vi "Configure Raw Frames RTM.vi"(8 "error in (no error)":errorcluster, 11 "Node Ptr":u64 format="%.0x") -> (0 "error out":errorcluster)   [LabVIEW 2020, in "AIM ARINC 664 System Explorer.lvlib" / "Implementation.lvlib"]
uses:
  Implementation.lvlib
  Frame Configuration/FrameEditor.lvlib
  Scripting/AIM ARINC 664 Scripting.lvlib
  <vilib>/Utility/SystemLogging/NI_SystemLogging.lvlib
  <vilib>/NI VeriStand/Custom Device Tools/Custom Device Utility Library/Custom Device Utility Library.lvlib
  <vilib>/NI VeriStand/Custom Device API/Custom Device API.lvlib
panel:
  in  "Tag":string
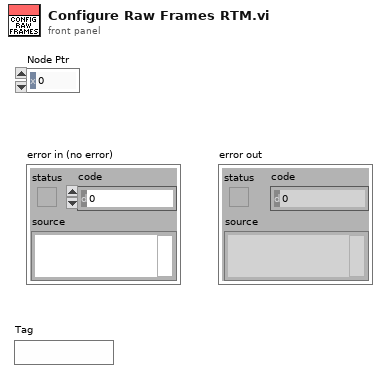
[diagram p1: front panel]
types:
  T1 = typedef "frame_record_type.ctl" = cluster{"HeaderInfo":T2, "Data":u8[]}
  T2 = typedef "AIM664LV.lvlib/queue_header_generic.ctl" = cluster{"InterFrameGap":u32, "PacketGroupWaitTime":u32, "PayloadBufferMode":u8, "PayloadGenerationMode":u8, "PreambleCount":u8, "Skew":u32, "NetSelect":u8, "FrameStartMode":u8, "PhysErrorInjection":u32, "SequenceNumberInit":u16, "SequenceNumberOffset":u16}
  T3 = typedef "Custom Device API.lvlib/Custom Device Item Ref.ctl" = u64
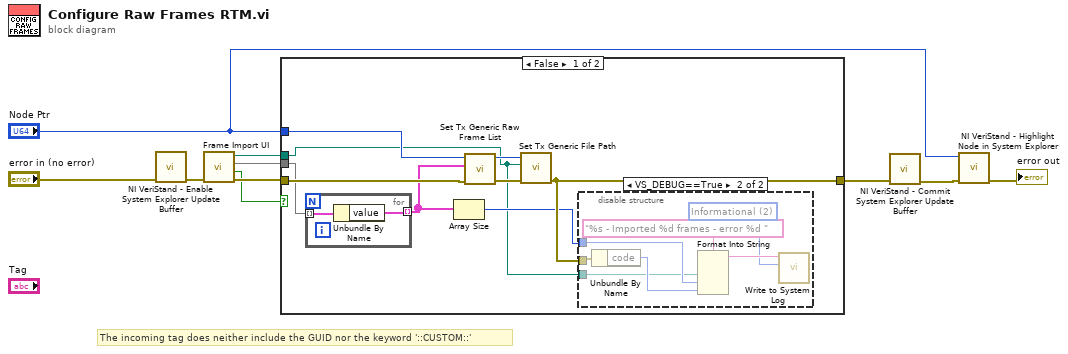
[diagram p0: block diagram]
diagram:
  # "The incoming tag does neither include the GUID nor the keyword '::CUSTOM::'"
  n1 = call <vilib>:"NI VeriStand - Enable System Explorer Update Buffer.vi"("error in (no error)"="error in (no error)") -> ("error out"=w2:errorcluster)  [unwired: 10 in]
  n2 = call "Frame Import UI.vi"("error in"=w2) -> ("error out"=w10:errorcluster, "Cancelled"=w9:bool, "frame map out"=w8:map{string, T1}, "Currently Loaded file"=w7:path)  [unwired: 7 in]
  n3 = case shown="False" w9 {
    tunnel: w10 -> [w16 w29]
    tunnel: [w13 w29] -> w5
    tunnel: "Node Ptr" -> [w18 _]
    tunnel: w8 -> [w15 _]
    tunnel: w7 -> [w11 _]
    frame False {
      n4 = for {
        tunnel: w15 -> [w28] mode=indexing
        tunnel: [w27] -> w14 mode=indexing
        n5 = Unbundle By Name(w28) -> ("value"=w27:T1)
      }
      n6 = Array Size(array=w14) -> (size(s)=w12:i32)
      n7 = call "Set Tx Generic Raw Frame List.vi"("error in"=w16, "Raw Frame List"=w14, "generic tx section in"=w18) -> ("error out"=w19:errorcluster, "generic tx section out"=w17:T3)  [unwired: 7 in]
      n8 = call "Set Tx Generic File Path.vi"("error in"=w19, "Frame Array File Path"=w11, "generic tx section in"=w17) -> ("error out"=w13:errorcluster)  [unwired: 7 in, 1 out]
      n9 = disable-structure shown="VS_DEBUG==True" {
        disable-tunnel: w13 -> [_ w23]
        disable-tunnel: w12 -> [_ w21]
        disable-tunnel: w11 -> [_ w20]
        frame condition #0 (active) {
        }
        frame condition #1 {
          w24 = 2 items=["Error", "Warning", "Informational"] ("severity")
          n10 = Unbundle By Name(w23) -> ("code"=w22:i32)
          n11 = Format Into String(format string="%s - Imported %d frames - error %d ", w20, w21, w22) -> (resulting string=w25:string)  [unwired: 2 in, 1 out]
          n12 = call <vilib>:"Write to System Log.vi"("severity"=w24, "message"=w25) -> ()  [unwired: 9 in, 1 out]
        }
      }
    }
    frame True {
    }
  }
  n13 = call <vilib>:"NI VeriStand - Commit System Explorer Update Buffer.vi"("error in (no error)"=w5) -> ("error out"=w4:errorcluster)  [unwired: 10 in]
  n14 = call <vilib>:"NI VeriStand - Highlight Node in System Explorer.vi"("error in (no error)"=w4, "Item Ref in"="Node Ptr") -> ("error out"=→"error out":errorcluster)  [unwired: 8 in, 1 out]
